vi "Configure Sequencer Trigger Timeout.vi"(8 "error in (no error)":errorcluster, 9 "Trigger Timeout (1.0)":dbl=1.0 format="%^.3e", 10 "Instance (1)":i32=1, 11 "VISA resource name":refnum<visa-resource-name>) -> (0 "error out":errorcluster, 3 "VISA resource name out":refnum<visa-resource-name>)   [LabVIEW 2020, in "Rohde&Schwarz CMXP GPRF.lvlib"]
doc: "Sets a timeout for waiting for a trigger event for List Increment = MEASUREMENT and TRIGGER.\n\nAttribute:\nRSCMXPGPRF_ATTR_SEQUENCER_TRIGGER_TIMEOUT\n\nRemote-control command:\nTRIGger:GPRF:GEN<i>:SEQuencer:TOUT"
uses:
  <instrlib>/Rohde&Schwarz CMXP GPRF/Rohde&Schwarz CMXP GPRF.lvlib
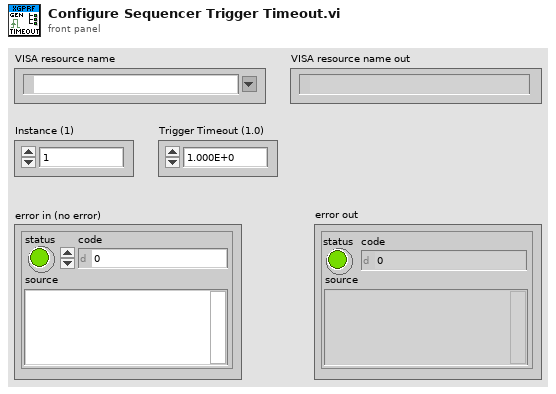
[diagram p1: front panel]
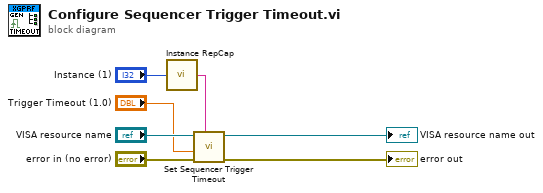
[diagram p0: block diagram]
diagram:
  n1 = call <instrlib>:"Instance RepCap.vi"("Instance in"="Instance (1)") -> ("Instance out"=w2:string)
  n2 = call "Set Sequencer Trigger Timeout"("Repeated Capabilities"=w2, "error in (no error)"="error in (no error)", "Sequencer Trigger Timeout (0.0)"="Trigger Timeout (1.0)", "instrument handle"="VISA resource name") -> ("error out"=→"error out":errorcluster, "instrument handle out"=→"VISA resource name out":refnum<visa-resource-name>)  [unwired: 6 in]
